vi "OCU_Main.vi"() -> ()   [LabVIEW 2013]
doc: "To be executed on the Opperator Control Unit (laptop), which communicates to a variety of platforms for the sailbot boat to send missions to complete, override commands, and to monitor the status of the boat and parts of the code run on it. It should be run in parallel with \"Main.vi\" in the cRIO code foler. \n\nCreaded by Victoria Coleman and Elizabeth Mahon (03/14)"
uses:
  cRIO_Code/Data/TypeDefs/MissionTypeControl.ctl
  cRIO_Code/Data/TypeDefs/UTM Location.ctl
  cRIO_Code/Data/TypeDefs/MissionDescription.ctl
  cRIO_Code/Data/TypeDefs/MainsailPositionIndicator.ctl
  cRIO_Code/Data/TypeDefs/JibPositionIndicator.ctl
  cRIO_Code/Data/TypeDefs/Rudder Set Suggestions.ctl
  cRIO_Code/Data/TypeDefs/OverrideMode.ctl
  cRIO_Code/Data/TypeDefs/Constants for OCU Tuning.ctl
  cRIO_Code/Data/TypeDefs/MotorSetup.ctl
  cRIO_Code/Data/TypeDefs/DynamixelSetupInfo.ctl
  TypeDef/map_list.ctl
  cRIO_Code/Data/TypeDefs/Sail Set Suggestions.ctl
  cRIO_Code/Data/TypeDefs/Sim_Wind_Heading.ctl
  cRIO_Code/Data/TypeDefs/Sim_Wind_Speed.ctl
  cRIO_Code/Logic/Classes/Missions/GenericMission/GenericMission.lvclass
  cRIO_Code/Data/TypeDefs/OverrideInformation.ctl
  cRIO_Code/Data/TypeDefs/Apparent Wind Point of Sail.ctl
  cRIO_Code/Data/TypeDefs/ObstacleDescription.ctl
  cRIO_Code/Logic/Classes/Obstacle/Obstacle.lvclass
  cRIO_Code/Data/TypeDefs/BoatType.ctl
  cRIO_Code/Logic/Classes/Waypoint/Waypoint.lvclass
  CommandMessages.ctl
  <vilib>/event_ctls.llb/eventvkey.ctl
  cRIO_Code/Logic/Classes/Missions/GoTo/GoTo.lvclass
  RIO-OCU_Comm/NetworkStreams/Writer/NetworkStreamWriter.lvclass
  RIO-OCU_Comm/NetworkStreams/Reader/NetworkStreamReader.lvclass
panel:
  in  "Do \"Initialize Me!\" Before running":enum32{"Initialize Me!", "Tuneable Constants"}(tab)
  in  "Boat Type":T1=enum."Damn Yankee"
  in  "Map":T2=enum."Olin"
  out "Writter\nConnected?":bool
  out "Reader\nConnected?":bool
  in  "OCU Tuning Constants":T3={"Motor Setting Constant"={"Main Dynamixel Set Data"={"Lower Winch Bound (deg)"=0.0, "Upper Winch Bound (deg)"=1000.0}, "Rudder Dynamixel Set Data"={"Lower Winch Bound (deg)"=30.0, "Upper Winch Bound (deg)"=90.0}, "Jib Dynamixel Set Data"={"Lower Winch Bound (deg)"=0.0, "Upper Winch Bound (deg)"=700.0}}, "Irons Range (deg)"=45.0}
  in  "Main Tab Structure":T6(tab)
  in  "Trace Path":bool=TRUE
  in  "Setting Missions with Map Internal Tab":T7(tab)
  in  "ClearMissionPOI":bool
  in  "CreateMission":bool
  in  "Mission Type":T8=enum."Drive to Waypoint"
  in  "Mission Points of Interest":T9[](array[typedef]) {"North" format="%#_10f"; "East" format="%#_8f"}
  in  "Tolerance (m)":dbl=10.0
  in  "Duration (s)\n[For in-box mission]":dbl=-1.0
  in  "Timeout (s)":dbl=-1.0
  out "Current Missions str":T10[](array[typedef]) {"Points of Interest"."North" format="%#_10f"; "Points of Interest"."East" format="%#_8f"}
  in  "ID# To Delete (miss)":u16
  in  "DeleteMission":bool
  out "# of Missions":i32
  in  "ClearObstaclePOI":bool
  out "# of Obstacles":i32
  in  "DeleteObstacle":bool
  in  "ID# To Delete (obs)":u16
  in  "Obstacle Points of Interest":T9[](array[typedef]) {"North" format="%#_10f"; "East" format="%#_8f"}
  in  "CreateObstacle":bool
  out "Current Obstacles":T11[](array[typedef]) {"Obstacle Array"."North" format="%#_10f"; "Obstacle Array"."East" format="%#_8f"}
  out "Robot Location":T9 {"North" format="%#_10f"; "East" format="%#_8f"}
  out "Rudder Setpoint":T12 min=-0.95 max=0.95 scale=1.0..-1.0
  out "BoatSpeed":dbl
  out "Abs Wind Direction":dbl(knob)
  out "Main":T13
  out "Jib":T14
  out "BoatDirection":dbl(knob)
  out "Rudder\noverridden?":bool
  out "Sail\noverridden?":bool
  out "RelWindDirection":T15 scale=0.0..360.0 scale format="%4d"
  in  "Sim_Wind_Heading":T16
  in  "Sim_Wind_Speed":T17
  out "Set Mission with Map":T18(plugin-control)
  in  "Clear Trace":bool
  in  "Plot Obstacles":bool=TRUE
  out "Sending IDs?":bool
  out "Manual Control Map":T18(plugin-control)
  in  "Main":T13
  in  "Jib":T14
  in  "Manual Rudder Setpoint":T12 min=-0.95 max=0.95 scale=1.0..-1.0
  in  "OverrideMode":T19
  out "Reset missions?":bool=TRUE
  out "Missions from Main":refnum<class "GenericMission.lvclass">[](array[class])
  out "Current Obstacles":refnum<class "Obstacle.lvclass">[](array[class])
  out "Current Missions":refnum<class "GenericMission.lvclass">[](array[class])
  out "Finished Missions":refnum<class "GenericMission.lvclass">[](array[class])
  out "Map display loop counter":i32
  out "User input loop counter":i32
  out "Desired Heading":dbl
  out "Abs Wind Direction":dbl(knob)
  out "Rel Wind Direction":dbl(knob)
  out "Sail Positions":T20 {"MainSailSuggestion" min=0.0 max=1.0; "JibSailSuggestion" min=0.0 max=1.0}
  out "Rudder Setpoint":T12 min=-0.95 max=0.95 scale=1.0..-1.0
  out "BoatDirection":dbl
  out "Override info":T21 {"SailSetting"."MainSailSuggestion" min=0.0 max=1.0; "SailSetting"."JibSailSuggestion" min=0.0 max=1.0; "Rudder Setpoint" min=-0.95 max=0.95 scale=1.0..-1.0}
  out "Final error out":errorcluster
  out "Intermediate\nWaypoints":refnum<class "Waypoint.lvclass">[](array[class])
  in  "stop":bool
  # "RUN MAIN.VI FIRST. SERIOUSLY"
  # "Add the \"Local GPS\" section of the old code so that we can grab GPS points from the boat and save them as waypoints or points of interest."
  # "If you forgot to set the boat type, you must restart the code"
  # "Reorganize this section, maybe split the cluster up"
  # "# of Waypoints Total [implement this]"
  # "# of Waypoints Left [implement this]"
  # "Log Message [important that we implement this one]"
  # "This is where you should be able to clilck the map and set a waypoint. Look in the [Mission Map] [Mission Edit]tab in the old OCU\n(\\Software\\0-OCU\\0 Code\\0 OCU.vi)\nand check out how they set up and documented the point and click operation.\nEric, 4/5/14"
  # "Add Load MDF, Save MDF, and Clear Mission functionality. Clear missions would clear all current missions. Look at old OCU for examples"
  # "This is where you should be able to clilck the map and set a waypoint. Look in the [Mission Map] [Mission Edit]tab in the old OCU\n(\\Software\\0-OCU\\0 Code\\0 OCU.vi)\nand check out how they set up and documented the point and click operation.\nEric, 4/5/14"
  # "Add Load ODF, Save ODF, and Clear Mission functionality. Clear missions would clear all current missions. Look at old OCU for examples"
  # "Look in the [Mission Map][Monitering]tab in the old OCU\n(\\Software\\0-OCU\\0 Code\\0 OCU.vi)\nand check out how they displayed the boat information during runtime. Try and make the indicators pretty and try to give only critical information \n\nEric, 4/5/14"
  # "Boat Direction\nis in \"math\"\n0E, CCW\nincrease"
  # "Abs Wind\nis in \"math\"\n0E, CCW\nincrease"
  # "Set wind speed"
  # "Set water current speed"
  # "Look in the lower right of the old OCU\n(\\Software\\0-OCU\\0 Code\\0 OCU.vi)\nand check out how they tweaked the simulator during runtime. Do this later.\n\nEric, 4/5/14"
  # "Set boat position"
  # "KEY MAPPINGS TO ACTUATOR MOVEMENT:\n\n\"Up\" -- Main out    |  \"Page Down\" -- Jib out\n\"Down\" -- Main in  |  \"Right\" -- Jib in\n\n\"Page Up\" -- rudder right\n\"Left\" -- rudder left"
  # "PUT MAP HERE"
  # "Check out the Manual Mission Input in the bottom left of the old code: (\\Software\\0-OCU\\0 Code\\0 OCU.vi)"
  # "PUT ALL THE BOAT DATA HERE\nLook at the Detailed Telemetry section of the old OCU for inspiration on how to organize information (\\Software\\0-OCU\\0 Code\\0 OCU.vi)"
  # "These guys need to be kept even though they aren't human readable, they're used for probing and data passage"
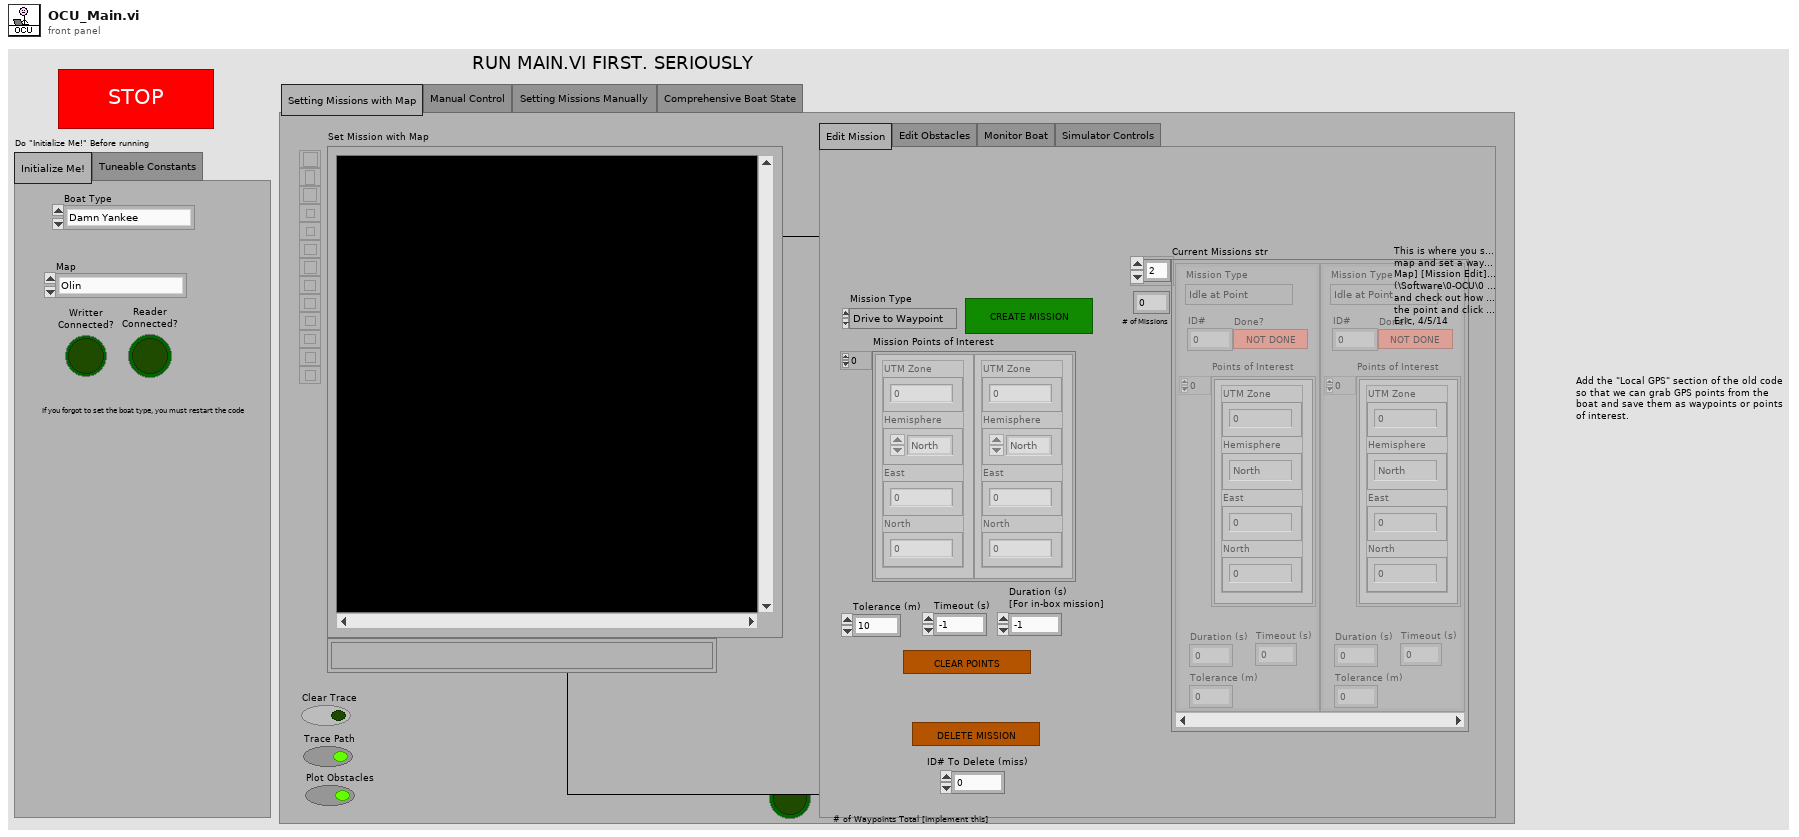
[diagram p1: front panel]
types:
  T1 = typedef "BoatType.ctl" = enum16{"Blackbody Radiation", "ReadLog", "Little boats", "Damn Yankee"}
  T2 = typedef "map_list.ctl" = enum16{"Grid", "Olin"}
  T3 = typedef "Constants for OCU Tuning.ctl" = cluster{"Motor Setting Constant":T4, "Irons Range (deg)":dbl}
  T4 = typedef "MotorSetup.ctl" = cluster{"Main Dynamixel Set Data":T5, "Rudder Dynamixel Set Data":T5, "Jib Dynamixel Set Data":T5}
  T5 = typedef "DynamixelSetupInfo.ctl" = cluster{"Lower Winch Bound (deg)":dbl, "Upper Winch Bound (deg)":dbl}
  T6 = enum32{"Setting Missions with Map", "Manual Control", "Setting Missions Manually ", "Comprehensive Boat State"}
  T7 = enum32{"Edit Mission", "Edit Obstacles", "Monitor Boat", "Simulator Controls"}
  T8 = typedef "MissionTypeControl.ctl" = enum16{"Idle at Point", "Drive to Waypoint", "Round Buoy to Port", "Round Buoy to Starboard", "Pass Between Buoys", "Station Keeping"}
  T9 = typedef "UTM Location.ctl" = cluster{"UTM Zone":dbl, "Hemisphere":enum16{"North", "South"}, "East":dbl, "North":dbl}
  T10 = typedef "MissionDescription.ctl" = cluster{"Duration (s)":dbl, "Timeout (s)":dbl, "Tolerance (m)":dbl, "Mission Type":T8, "Points of Interest":T9[], "ID#":i32, "Done?":bool}
  T11 = typedef "ObstacleDescription.ctl" = cluster{"ID#":i32, "Obstacle Array":T9[]}
  T12 = typedef "Rudder Set Suggestions.ctl" = dbl
  T13 = typedef "MainsailPositionIndicator.ctl" = dbl
  T14 = typedef "JibPositionIndicator.ctl" = dbl
  T15 = typedef "Apparent Wind Point of Sail.ctl" = dbl
  T16 = typedef "Sim_Wind_Heading.ctl" = dbl
  T17 = typedef "Sim_Wind_Speed.ctl" = dbl
  T18 = typedef "IMAQ Image.ctl" = refnum<image>
  T19 = typedef "OverrideMode.ctl" = enum16{"None", "Rudder", "Sails", "Both"}
  T20 = typedef "Sail Set Suggestions.ctl" = cluster{"MainSailSuggestion":dbl, "JibSailSuggestion":dbl}
  T21 = typedef "OverrideInformation.ctl" = cluster{"OverrideMode":T19, "SailSetting":T20, "Rudder Setpoint":T12, "Sim_Wind_Speed":dbl, "Sim_Wind_Heading":dbl}
  T22 = typedef "mission_arrays.ctl" = cluster{"# of Missions":i32, "Readable Missions":T10[], "Mission array":refnum<class "GenericMission.lvclass">[]}
  T23 = typedef "obstacle_arrays.ctl" = cluster{"# of Obstacles":i32, "Obstacle array":refnum<class "Obstacle.lvclass">[], "Readable Obstacles":T11[]}
  T24 = typedef "map_metadata.ctl" = cluster{"Meters/pixel":dbl, "Top Left Pixel UTM":T9, "Bottom Right Pixel UTM":T9}
  T25 = typedef "CommandMessages.ctl" = enum16{"Pass", "OverrideMode", "Add mission", "Delete mission", "Add obstacle", "Delete obstacle", "Change constants", "Check mission ID", "Check obstacle ID"}
  T26 = typedef "eventvkey.ctl" = enum16{"ASCII", "Enter", "Return", "Shift", "Ctrl", "Alt", "Cmd", "Opt", "Caps", "NumLock", "Clear", "Break", "Up", "Down", "Left", "Right", "Insert", "Delete", "Home", "End", "PageUp", "PageDown", "Escape", "Help", "Pause", "ScrollLock", "F1", "F2", "F3", "F4", "F5", "F6", "F7", "F8", "F9", "F10", "F11", "F12", "F13", "F14", "F15", "F16", "F17", "F18", "F19", "F20", "F21", "F22", "F23", "F24", "Play", "VolumeUp", "VolumeDown", "Mute", "Two Byte Char"}
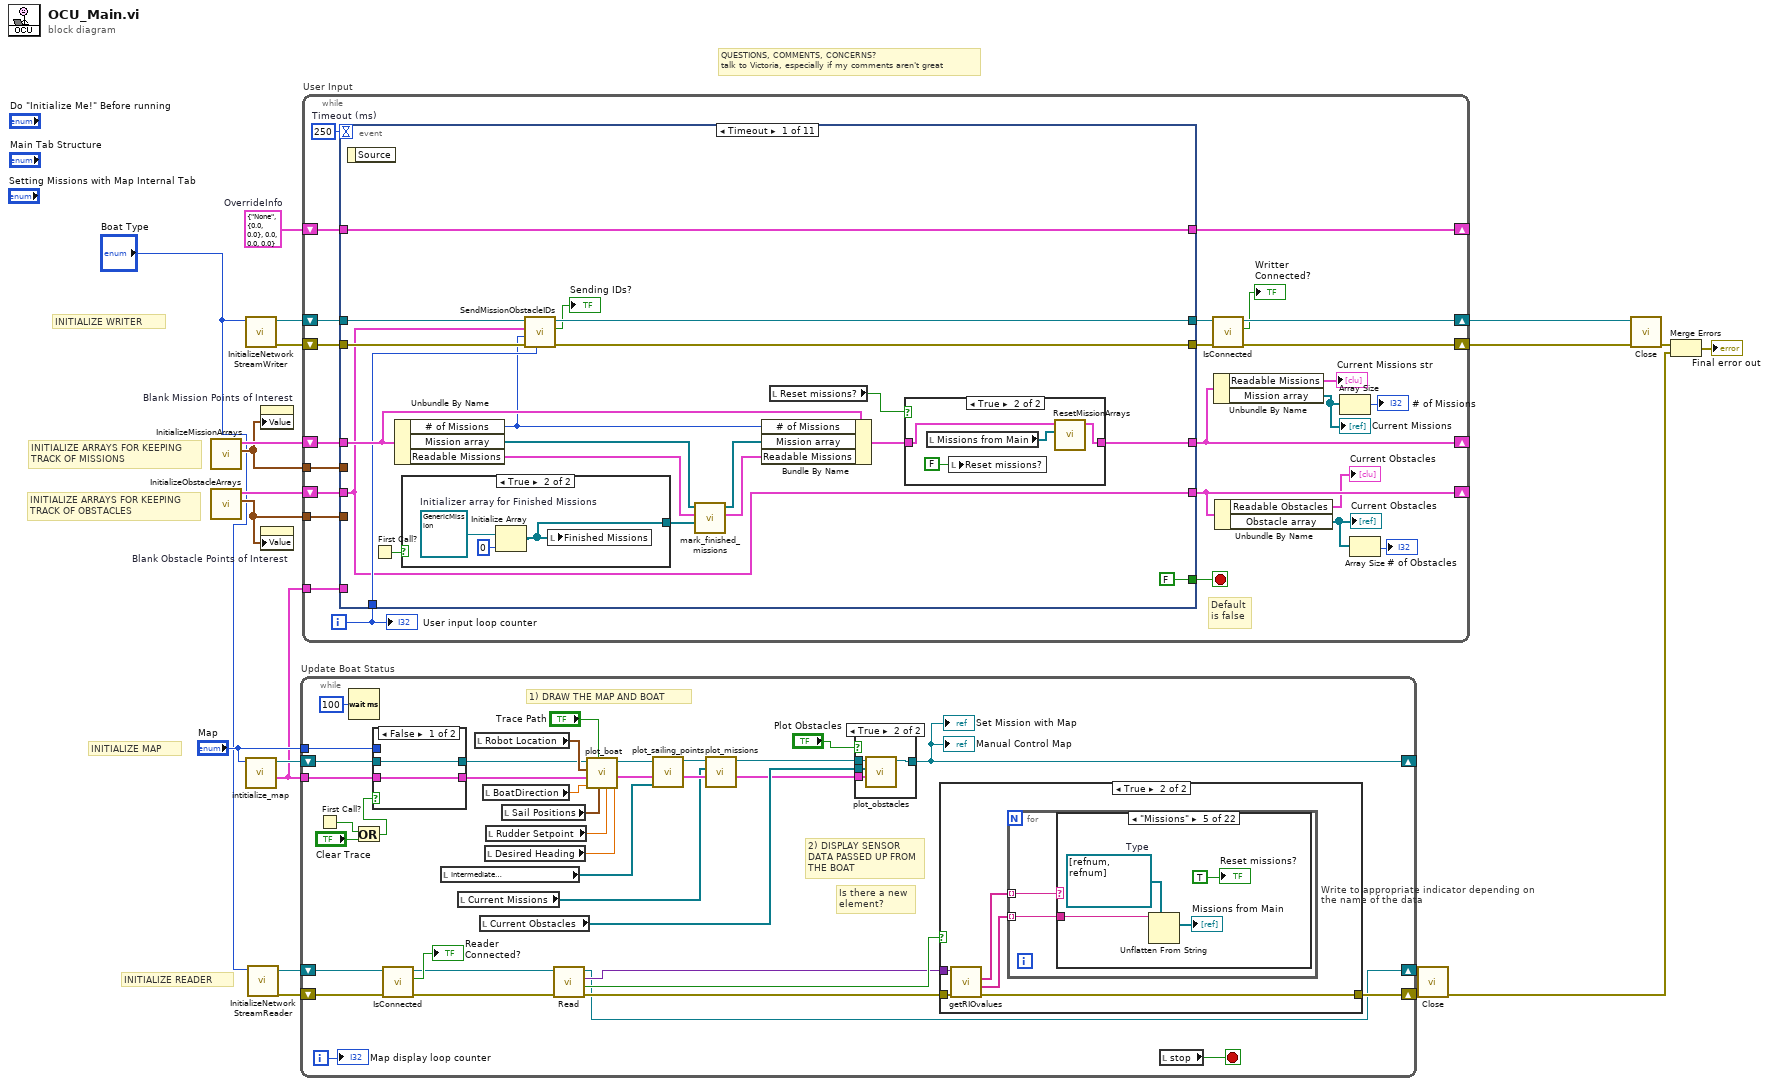
[diagram p0: block diagram]
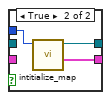
[diagram p3: hidden frame]
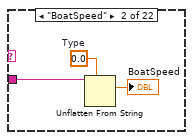
[diagram p6: hidden frame]
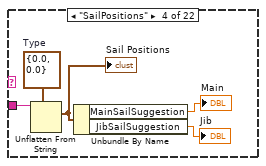
[diagram p8: hidden frame]
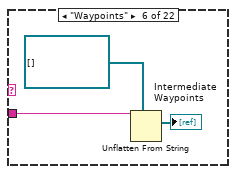
[diagram p9: hidden frame]
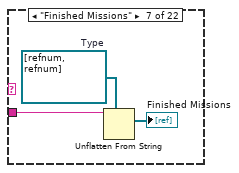
[diagram p10: hidden frame]
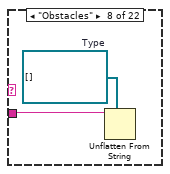
[diagram p11: hidden frame]
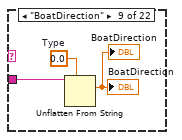
[diagram p12: hidden frame]
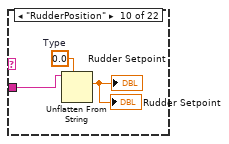
[diagram p13: hidden frame]
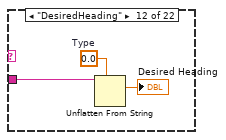
[diagram p15: hidden frame]
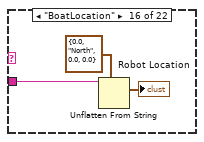
[diagram p19: hidden frame]
diagram:
  w6 = T21 {"OverrideMode"=enum."None", "SailSetting"={"MainSailSuggestion"=0.0, "JibSailSuggestion"=0.0}, "Rudder Setpoint"=0.0, "Sim_Wind_Speed"=0.0, "Sim_Wind_Heading"=0.0}  # OverrideInfo
  # "INITIALIZE ARRAYS FOR KEEPING TRACK OF OBSTACLES"
  # "INITIALIZE WRITER"
  # "INITIALIZE ARRAYS FOR KEEPING TRACK OF MISSIONS"
  # "INITIALIZE MAP"
  # "INITIALIZE READER"
  # "QUESTIONS, COMMENTS, CONCERNS? \ntalk to Victoria, especially if my comments aren't great"
  n1 = call "InitializeMissionArrays.vi"() -> ("Mission Points of Interest"=w2:T9[], "Initialized Mission Arrays"=w20:T22)  [unwired: 10 in]
  n2 = call "InitializeObstacleArrays.vi"() -> ("Obstacle Points of Interest"=w3:T9[], "Obstacle Arrays Cluster"=w4:T23)  [unwired: 10 in]
  n3 = call "InitializeNetworkStreamWriter.vi"("Boat Type"="Boat Type") -> ("error out"=w17:errorcluster, "NetworkStreamWriter out"=w16:refnum<class "NetworkStreamWriter.lvclass">)  [unwired: 9 in]
  n4 = call "intitialize_map.vi"("Map"="Map") -> ("MapDistanceInfo"=w5:T24, "Map Image Out"=w13:T18)  [unwired: 9 in]
  n5 = call "InitializeNetworkStreamReader.vi"("Boat Type"="Boat Type") -> ("error out"=w11:errorcluster, "NetworkStreamReader out"=w12:refnum<class "NetworkStreamReader.lvclass">)  [unwired: 9 in]
  n6 = property on="Blank Mission Points of Interest" class="Arr (strict)"("Value"=w2) -> ()  [unwired: 2 in, 2 out]
  n7 = property on="Blank Obstacle Points of Interest" class="Arr (strict)"("Value"=w3) -> ()  [unwired: 2 in, 2 out]
  n8 = while "Update Boat Status" {
    shift-right: [w47] -> w15
    shift-left: w12 -> [w57]
    shift-right: [w53] -> w14
    shift-left: w11 -> [w56]
    tunnel: w5 -> [w42]
    tunnel: "Map" -> [w44]
    shift-right: [w29] -> _
    shift-left: w13 -> [w45]
    i -> [w43]
    stop <- w58 stop-if-true
    # "Is there a new element?"
    # "2) DISPLAY SENSOR DATA PASSED UP FROM THE BOAT"
    # "1) DRAW THE MAP AND BOAT"
    n9 = First Call?() -> (First Call?: T/F=w32:bool)
    n10 = Wait (ms)(milliseconds to wait=u32 100) -> ()  [unwired: 1 out]
    n11 = Or(x=w32, y="Clear Trace") -> (x .or. y?=w31:bool)
    n12 = case shown="False" w31 {
      tunnel: w45 -> [w65 _]
      tunnel: [w65 w66] -> w34
      tunnel: w42 -> [w64 _]
      tunnel: [w64 w67] -> w35
      tunnel: w44 -> [_ w68]
      frame False {
      }
      frame True {
        n13 = call "intitialize_map.vi"("Map"=w68) -> ("MapDistanceInfo"=w67:T24, "Map Image Out"=w66:T18)  [unwired: 9 in]
      }
    }
    n14 = call "IsConnected.vi"("error in (no error)"=w56, "NetworkStreamReader in"=w57) -> ("error out"=w51:errorcluster, "Connected?"=→"Reader\nConnected?":bool, "NetworkStreamReader out"=w52:refnum<class "NetworkStreamReader.lvclass">)  [unwired: 7 in]
    n15 = local read "Intermediate\nWaypoints"() -> (w26:refnum<class "Waypoint.lvclass">[])
    n16 = local read "Current Missions"() -> (w21:refnum<class "GenericMission.lvclass">[])
    n17 = local read "Robot Location"() -> (w38:T9)
    n18 = local read "Current Obstacles"() -> (w28:refnum<class "Obstacle.lvclass">[])
    n19 = local read "BoatDirection"() -> (w40:dbl)
    n20 = local read "Desired Heading"() -> (w30:dbl)
    n21 = local read "Rudder Setpoint"() -> (w39:T12)
    n22 = local read "Sail Positions"() -> (w41:T20)
    n23 = call "Read.vi"("error in (no error)"=w51, "NetworkStreamReader in"=w52) -> ("error out"=w50:errorcluster, "New element?"=w49:bool, "element"=w48:variant, "NetworkStreamReader out"=w47:refnum<class "NetworkStreamReader.lvclass">)  [unwired: 5 in, 1 out]
    n24 = call "plot_boat.vi"("Desired Heading"=w30, "Rudder Setpoint"=w39, "Sail Setpoints"=w41, "Trace Path"="Trace Path", "Heading"=w40, "MapDistanceInfo"=w35, "UTM Location"=w38, "Map in"=w34) -> ("MapDistanceInfo OUT"=w36:T24, "Map Out"=w37:T18)  [unwired: 1 in, 1 out]
    n25 = call "plot_sailing_points.vi"("Intermediate\nWaypoints"=w26, "MapDistanceInfo"=w36, "Map in"=w37) -> ("MapDistanceInfo OUT"=w25:T24, "Map Out"=w23:T18)  [unwired: 6 in, 1 out]
    n26 = call "plot_missions.vi"("MapDistanceInfo"=w25, "Missions"=w21, "Map in"=w23) -> ("MapDistanceInfo OUT"=w24:T24, "Map Out"=w22:T18)  [unwired: 6 in, 1 out]
    n27 = case shown="True" "Plot Obstacles" {
      tunnel: w22 -> [w59 w63]
      tunnel: [w59 w62] -> w29
      tunnel: w24 -> [_ w61]
      tunnel: w28 -> [_ w60]
      frame False {
      }
      frame True {
        n28 = call "plot_obstacles.vi"("MapDistanceInfo"=w61, "Current Obstacles"=w60, "Map in"=w63) -> ("Map Out"=w62:T18)  [unwired: 7 in, 1 out]
      }
    }
    "Set Mission with Map" <- w29
    "Manual Control Map" <- w29
    n29 = case shown="True" w49 {
      tunnel: [w69 w72] -> w53
      tunnel: w50 -> [w69 w71]
      tunnel: w48 -> [_ w70]
      frame False {
      }
      frame True {
        n30 = call "getRIOvalues.vi"("error in"=w71, "element"=w70) -> ("error out"=w72:errorcluster, "data"=w73:string[], "names"=w74:string[])  [unwired: 7 in]
        n31 = for "Write to appropriate indicator depending on the name of the data" {
          tunnel: w74 -> [w76] mode=indexing
          tunnel: w73 -> [w75] mode=indexing
          n32 = case shown="\"Missions\"" w76 {
            tunnel: w75 -> [_ w77 _ w84 w87 w91 w94 w95 w99 w102 _ w103 _ _ _ w108 _ _ _ w110 w114 _]
            frame Default {
              # "unknown name"
            }
            frame "BoatSpeed" {
              w79 = 0.0  # Type
              n33 = Unflatten From String(type=w79, binary string=w77) -> (value=→"BoatSpeed":dbl)  [unwired: 3 in, 2 out]
            }
            frame "WindSpeed" {
            }
            frame "SailPositions" {
              w83 = T20 {"MainSailSuggestion"=0.0, "JibSailSuggestion"=0.0}  # Type
              n34 = Unflatten From String(type=w83, binary string=w84) -> (value=w82:T20)  [unwired: 3 in, 2 out]
              "Sail Positions" <- w82
              n35 = Unbundle By Name(w82) -> ("MainSailSuggestion"=→"Main":dbl, "JibSailSuggestion"=→"Jib":dbl)
            }
            frame "Missions" {
              w88 = refnum<class "GenericMission.lvclass">[] [refnum, refnum]  # Type
              n36 = Unflatten From String(type=w88, binary string=w87) -> (value=→"Missions from Main":refnum<class "GenericMission.lvclass">[])  [unwired: 3 in, 2 out]
              "Reset missions?" <- TRUE
            }
            frame "Waypoints" {
              n37 = Unflatten From String(type=refnum<class "Waypoint.lvclass">[] [] ("elements"), binary string=w91) -> (value=→"Intermediate\nWaypoints":refnum<class "Waypoint.lvclass">[])  [unwired: 3 in, 2 out]
            }
            frame "Finished Missions" {
              w93 = refnum<class "GenericMission.lvclass">[] [refnum, refnum]  # Type
              n38 = Unflatten From String(type=w93, binary string=w94) -> (value=→"Finished Missions":refnum<class "GenericMission.lvclass">[])  [unwired: 3 in, 2 out]
            }
            frame "Obstacles" {
              w96 = refnum<class "Obstacle.lvclass">[] []  # Type
              n39 = Unflatten From String(type=w96, binary string=w95) -> ()  [unwired: 3 in, 3 out]
            }
            frame "BoatDirection" {
              w98 = 0.0  # Type
              n40 = Unflatten From String(type=w98, binary string=w99) -> (value=→"BoatDirection" →"BoatDirection":dbl)  [unwired: 3 in, 2 out]
            }
            frame "RudderPosition" {
              w101 = T12 0.0  # Type
              n41 = Unflatten From String(type=w101, binary string=w102) -> (value=→"Rudder Setpoint" →"Rudder Setpoint":T12)  [unwired: 3 in, 2 out]
            }
            frame "SimWindSpeed(m/s)" {
            }
            frame "DesiredHeading" {
              w105 = 0.0  # Type
              n42 = Unflatten From String(type=w105, binary string=w103) -> (value=→"Desired Heading":dbl)  [unwired: 3 in, 2 out]
            }
            frame "RudderForce" {
            }
            frame "BatteryVoltage" {
            }
            frame "StayForces" {
            }
            frame "BoatLocation" {
              n43 = Unflatten From String(type=T9 {"UTM Zone"=0.0, "Hemisphere"=enum."North", "East"=0.0, "North"=0.0} ("UTM Location"), binary string=w108) -> (value=→"Robot Location":T9)  [unwired: 3 in, 2 out]
            }
            frame "Pitch" {
            }
            frame "Roll" {
            }
            frame "RateOfTurn" {
            }
            frame "RelWindDirection" {
              w111 = 0.0  # Type
              n44 = Unflatten From String(type=w111, binary string=w110) -> (value=→"Rel Wind Direction" →"RelWindDirection":dbl)  [unwired: 3 in, 2 out]
            }
            frame "AbsWindDirection" {
              w113 = 0.0  # Type
              n45 = Unflatten From String(type=w113, binary string=w114) -> (value=→"Abs Wind Direction" →"Abs Wind Direction":dbl)  [unwired: 3 in, 2 out]
            }
            frame "DynamixelTorques" {
            }
          }
        }
      }
    }
    n46 = local read "stop"() -> (w58:bool)
    "Map display loop counter" <- w43
  }
  n47 = while "User Input" {
    shift-right: [w124] -> _
    shift-left: w20 -> [w139]
    shift-right: [w132] -> w18
    shift-left: w17 -> [w136]
    shift-right: [w133] -> w19
    shift-left: w16 -> [w135]
    shift-right: [w130] -> _
    shift-left: w6 -> [w129]
    tunnel: w5 -> [w127]
    tunnel: w2 -> [w126]
    tunnel: w3 -> [w121]
    shift-right: [w119] -> _
    shift-left: w4 -> [w120]
    i -> [w115]
    stop <- w137 stop-if-true
    w125 = 250  # Timeout (ms)
    # "Default is false"
    n48 = event shown="[0] Timeout" {
      selector: _ -> [_ _ _ _ _ _ _ _ _ _ _]
      dyn-events: _ -> [_ _ _ _ _ _ _ _ _ _ _]
      timeout: w125 -> [_ _ _ _ _ _ _ _ _ _ _]
      tunnel: w139 -> [w155 w171 w189 w211 w236 w255 w262 w278 w290 w338 w369]
      tunnel: [FALSE TRUE FALSE _ FALSE _ _ _ _ _ _] -> w137
      tunnel: [w144 w170 w182 w212 w245 w253 w259 w273 w293 w336 w367] -> w128
      tunnel: w135 -> [w149 w173 w187 w215 w243 w251 w258 w276 w301 w357 w373]
      tunnel: w136 -> [w150 w170 w186 w214 w244 w254 w261 w281 w299 w347 w374]
      tunnel: [w145 w173 w185 w213 w242 w252 w258 w276 w300 w356 w372] -> w134
      tunnel: [w158 w172 w184 w218 w241 w256 w257 w279 w291 w342 w370] -> w130
      tunnel: w129 -> [w158 w172 w184 w218 w241 w256 w257 w279 w292 w355 w370]
      tunnel: w127 -> [_ _ _ _ _ _ _ w282 _ _ _]
      tunnel: w126 -> [_ _ w183 _ _ _ w265 _ _ _ _]
      tunnel: [w141 w171 w176 w211 w240 w255 w262 w278 w290 w338 w369] -> w124
      tunnel: w121 -> [_ _ _ w210 _ _ w264 _ _ _ _]
      tunnel: w120 -> [w147 w169 w175 w209 w239 w248 w263 w277 w289 w337 w368]
      tunnel: [w147 w169 w175 w208 w239 w247 w263 w277 w289 w337 w368] -> w119
      tunnel: w115 -> [w148 _ _ _ _ _ _ _ _ _ _]
      event Timeout {
        n49 = event-data() -> ()  [unwired: 1 in, 1 out]
        n50 = First Call?() -> (First Call?: T/F=w156:bool)
        n51 = Unbundle By Name(w155) -> ("# of Missions"=w146:i32, "Mission array"=w154:refnum<class "GenericMission.lvclass">[], "Readable Missions"=w153:T10[])
        n52 = case shown="True" w156 {
          tunnel: [w165 w166] -> w157
          frame False {
            n53 = local read "Finished Missions"() -> (w165:refnum<class "GenericMission.lvclass">[])
          }
          frame True {
            w168 = refnum<class "GenericMission.lvclass"> refnum  # Initializer array for Finished Missions
            n54 = Initialize Array(w168, 0 ("dimension size")) -> (w166:refnum<class "GenericMission.lvclass">[])
            n55 = local write "Finished Missions"(w166) -> ()
          }
        }
        n56 = call "SendMissionObstacleIDs.vi"("Loop counter"=w148, "error in (no error)"=w150, "# of Missions"=w146, "Obstacle Arrays Cluster"=w147, "NetworkStreamWriter in"=w149) -> ("error out"=w144:errorcluster, "Sending IDs?"=→"Sending IDs?":bool, "NetworkStreamWriter out"=w145:refnum<class "NetworkStreamWriter.lvclass">)  [unwired: 4 in]
        n57 = call "mark_finished_missions.vi"("Finished Missions"=w157, "Current Missions (human readable)"=w153, "Current Missions"=w154) -> (2:"Current Missions OUT"=w152:T10[], 3:"Current Missions OUT"=w151:refnum<class "GenericMission.lvclass">[])  [unwired: 7 in]
        n58 = Bundle By Name(cluster=w155, "# of Missions"=w146, "Mission array"=w151, "Readable Missions"=w152) -> (w142:T22)
        n59 = local read "Reset missions?"() -> (w143:bool)
        n60 = case shown="True" w143 {
          tunnel: w142 -> [w160 w163]
          tunnel: [w160 w162] -> w141
          frame False {
          }
          frame True {
            n61 = local read "Missions from Main"() -> (w161:refnum<class "GenericMission.lvclass">[])
            n62 = local write "Reset missions?"(FALSE ("Reset missions?")) -> ()
            n63 = call "ResetMissionArrays.vi"("Mission Array Replacement"=w161, "Mission Arrays"=w163) -> ("Mission Arrays"=w162:T22)  [unwired: 9 in]
          }
        }
      }
      event "stop": Value Change {
        # "Putting the button in here keeps the code from breaking, leave it here :)\nHas to do with how event structures work"
        n64 = event-data() -> ()  [unwired: 1 in, 2 out]
      }
      event "CreateMission": Value Change {
        n65 = event-data() -> ("OldVal"=w177:bool)  [unwired: 1 in]
        n66 = Array Size(array="Mission Points of Interest") -> (size(s)=w180:i32)
        n67 = Not Equal To 0?(x=w180) -> (x != 0?=w178:bool)
        n68 = And(x=w177, y=w178) -> (x .and. y?=w179:bool)
        n69 = case shown="False" w179 {
          tunnel: w189 -> [w190 w200]
          tunnel: [w190 w194] -> w176
          tunnel: [w192 w202] -> w182
          tunnel: w187 -> [w191 w205]
          tunnel: w186 -> [w192 _]
          tunnel: [w191 w203] -> w185
          tunnel: w183 -> [_ w193]
          tunnel: "Mission Points of Interest" -> [_ w199]
          frame False {
          }
          frame True {
            # "send created message to Forebrain"
            n70 = property on="Mission Points of Interest" class="Arr (strict)"("Value"=w193) -> ()  [unwired: 2 in, 2 out]
            n71 = call "CreateNewMissions.vi"("Timeout (s)"="Timeout (s)", "Duration (s)\n[For in-box mission]"="Duration (s)\n[For in-box mission]", "Tolerance (m)"="Tolerance (m)", "Mission Type"="Mission Type", "Points of Interest"=w199, "Initialized Mission Arrays"=w200) -> ("New Mission OUT"=w195:refnum<class "GenericMission.lvclass">, "Mission Array Cluster"=w194:T22)  [unwired: 4 in]
            n72 = Flatten To String(anything=w195) -> (data string=w204:string, error out=w201:errorcluster)  [unwired: 3 in, 1 out]
            n73 = call "MapAndWrite.vi"("error in (no error)"=w201, "String_Cast_of_Info"=w204, "Commands"=CommandMessages."Add mission", "NetworkStreamWriter in"=w205) -> ("error out"=w202:errorcluster, "NetworkStreamWriter out"=w203:refnum<class "NetworkStreamWriter.lvclass">)  [unwired: 2 in]
          }
        }
      }
      event "CreateObstacle": Value Change {
        n74 = event-data() -> ("OldVal"=w219:bool)  [unwired: 1 in]
        n75 = Array Size(array="Obstacle Points of Interest") -> (size(s)=w221:i32)
        n76 = Not Equal To 0?(x=w221) -> (x != 0?=w220:bool)
        n77 = And(x=w219, y=w220) -> (x .and. y?=w217:bool)
        n78 = case shown="True" w217 {
          tunnel: "Obstacle Points of Interest" -> [_ w229]
          tunnel: w215 -> [w224 w230]
          tunnel: w214 -> [w223 _]
          tunnel: [w224 w232] -> w213
          tunnel: [w223 w231] -> w212
          tunnel: w210 -> [_ w225]
          tunnel: w209 -> [w222 w228]
          tunnel: [w222 w227] -> w208
          frame False {
          }
          frame True {
            # "send created message to Forebrain"
            n79 = property on="Obstacle Points of Interest" class="Arr (strict)"("Value"=w225) -> ()  [unwired: 2 in, 2 out]
            n80 = call "CreateNewObstacles.vi"("Obstacle Arrays Cluster IN"=w228, "Points of Interest"=w229) -> ("Obstacle Arrays Cluster OUT"=w227:T23, "New Obstacle OUT"=w226:refnum<class "Obstacle.lvclass">)  [unwired: 8 in]
            n81 = Flatten To String(anything=w226) -> (data string=w234:string, error out=w233:errorcluster)  [unwired: 3 in, 1 out]
            n82 = call "MapAndWrite.vi"("error in (no error)"=w233, "String_Cast_of_Info"=w234, "Commands"=CommandMessages."Add obstacle", "NetworkStreamWriter in"=w230) -> ("error out"=w231:errorcluster, "NetworkStreamWriter out"=w232:refnum<class "NetworkStreamWriter.lvclass">)  [unwired: 2 in]
          }
        }
      }
      event "DeleteMission": Value Change {
        n83 = event-data() -> ("OldVal"=w238:bool)  [unwired: 1 in]
        n84 = call "DeleteMission.vi"("OldVal"=w238, "ID# To Delete (miss)"="ID# To Delete (miss)", "error in (no error)"=w244, "Initialized Mission Arrays in"=w236, "NetworkStreamWriter in"=w243) -> ("error out"=w245:errorcluster, "Initialized Mission Arrays out"=w240:T22, "NetworkStreamWriter out"=w242:refnum<class "NetworkStreamWriter.lvclass">)  [unwired: 4 in]
      }
      event "DeleteObstacle": Value Change {
        n85 = event-data() -> ("OldVal"=w249:bool)  [unwired: 1 in]
        n86 = call "DeleteObstacle.vi"("OldVal"=w249, "ID# To Delete (miss)"="ID# To Delete (obs)", "error in (no error)"=w254, "Obstacle Arrays Cluster IN"=w248, "NetworkStreamWriter in"=w251) -> ("error out"=w253:errorcluster, "Obstacle Arrays Cluster OUT"=w247:T23, "NetworkStreamWriter out"=w252:refnum<class "NetworkStreamWriter.lvclass">)  [unwired: 4 in]
      }
      event "ClearObstaclePOI", "ClearMissionPOI": Value Change {
        n87 = event-data() -> ()  [unwired: 1 in, 2 out]
        n88 = property on="Setting Missions with Map Internal Tab" class="TabCtl (strict)"(error in=w261) -> (error out=w260:errorcluster, "Value"=w266:T7)  [unwired: 1 in, 1 out]
        n89 = case shown="\"Edit Mission\", Default" w266 {
          tunnel: w265 -> [w269 _]
          tunnel: w264 -> [_ w272]
          tunnel: w260 -> [w268 w271]
          tunnel: [w267 w270] -> w259
          frame "Edit Mission", Default {
            n90 = property on="Mission Points of Interest" class="Arr (strict)"(error in=w268, "Value"=w269) -> (error out=w267:errorcluster)  [unwired: 1 in, 1 out]
          }
          frame "Edit Obstacles" {
            n91 = property on="Obstacle Points of Interest" class="Arr (strict)"(error in=w271, "Value"=w272) -> (error out=w270:errorcluster)  [unwired: 1 in, 1 out]
          }
        }
      }
      event "Set Mission with Map": Mouse Up {
        n92 = event-data() -> ()  [unwired: 1 in, 3 out]
        n93 = property on="Set Mission with Map" class="ImageControl"(error in=w281) -> (error out=w273:errorcluster, "Last Mouse Position"=w280:cluster{"X":i32, "Y":i32})  [unwired: 1 in, 1 out]
        n94 = call "ImageUTMPosition.vi"("Pixel Coordinates"=w280, "MapDistanceInfo"=w282) -> ("output cluster"=w274:T9)  [unwired: 9 in]
        n95 = property on="Setting Missions with Map Internal Tab" class="TabCtl (strict)"() -> ("Value"=w275:T7)  [unwired: 2 in, 2 out]
        n96 = case shown="\"Edit Obstacles\"" w275 {
          tunnel: w274 -> [_ w283 w286]
          frame Default {
          }
          frame "Edit Mission" {
            n97 = property on="Mission Points of Interest" class="Arr (strict)"() -> ("Value"=w284:T9[])  [unwired: 2 in, 2 out]
            n98 = Build Array (concatenate)(w284, w283) -> (w285:T9[])
            n99 = property on="Mission Points of Interest" class="Arr (strict)"("Value"=w285) -> ()  [unwired: 2 in, 2 out]
          }
          frame "Edit Obstacles" {
            n100 = property on="Obstacle Points of Interest" class="Arr (strict)"() -> ("Value"=w287:T9[])  [unwired: 2 in, 2 out]
            n101 = Build Array (concatenate)(w287, w286) -> (w288:T9[])
            n102 = property on="Obstacle Points of Interest" class="Arr (strict)"("Value"=w288) -> ()  [unwired: 2 in, 2 out]
          }
        }
      }
      event Key Down; Key Repeat {
        n103 = event-data() -> ("VKey"=w295:T26)  [unwired: 1 in]
        n104 = local read "OverrideMode"() -> (w294:T19)
        n105 = case "Only if Special key pressed" shown="Default" w295 {
          selector: w295 -> [_ w312]
          tunnel: w301 -> [w304 w309]
          tunnel: [w304 w310] -> w300
          tunnel: w299 -> [w303 w311]
          tunnel: [w303 w307] -> w293
          tunnel: "Manual Rudder Setpoint" -> [_ w315]
          tunnel: "Jib" -> [_ w314]
          tunnel: "Main" -> [_ w313]
          tunnel: w294 -> [_ w308]
          tunnel: w292 -> [w302 w306]
          tunnel: [w302 w305] -> w291
          frame "ASCII" {
            # "No special key pressed :("
          }
          frame Default {
            n106 = case "Only executes of any actuators are in override mode" shown="Default" w308 {
              selector: w308 -> [_ w319]
              tunnel: w315 -> [_ w333]
              tunnel: w314 -> [_ w334]
              tunnel: w313 -> [_ w335]
              tunnel: w312 -> [_ w332]
              tunnel: w311 -> [w317 w331]
              tunnel: [w318 w327] -> w310
              tunnel: w309 -> [w318 w328]
              tunnel: [w317 w329] -> w307
              tunnel: w306 -> [w316 w326]
              tunnel: [w316 w321] -> w305
              frame "None" {
              }
              frame Default {
                # "KEY MAPPINGS TO ACTUATOR MOVEMENT:\n\"Page Up\" -- rudder right       |    \"Up\" -- Main out          |     \"Page Down\" -- Jib out\n\"Left\" -- rudder left                  |      \"Down\" -- Main in     |      \"Right\" -- Jib in"
                n107 = call "Write_NetworkStream_OCU_Override.vi"("VKey"=w332, "Mainsail Position"=w335, "Jib Position"=w334, "Rudder Setpoint"=w333, "error in (no error)"=w331, "OverrideMode"=w319) -> ("Main Position"=w323:T13, "Jib Position"=w324:T14, "Rudder Position"=w325:T12, "error out"=w330:errorcluster)  [unwired: 5 in, 1 out]
                n108 = Bundle By Name(cluster=w326, "OverrideMode"=w319, "SailSetting.MainSailSuggestion"=w323, "SailSetting.JibSailSuggestion"=w324, "Rudder Setpoint"=w325) -> (w321:T21)
                n109 = Flatten To String(anything=w321) -> (data string=w322:string)  [unwired: 3 in, 2 out]
                n110 = call "MapAndWrite.vi"("error in (no error)"=w330, "String_Cast_of_Info"=w322, "Commands"=CommandMessages."OverrideMode", "NetworkStreamWriter in"=w328) -> ("error out"=w329:errorcluster, "NetworkStreamWriter out"=w327:refnum<class "NetworkStreamWriter.lvclass">)  [unwired: 2 in]
              }
            }
          }
        }
      }
      event Value Change {
        # "Just an obscure key to make everything update (hackish solution to reuse vi)"
        n111 = event-data() -> ()  [unwired: 1 in, 2 out]
        n112 = local read "Manual Rudder Setpoint"() -> (w350:T12)
        n113 = local read "Jib"() -> (w351:T14)
        n114 = local read "OverrideMode"() -> (w348:T19)
        n115 = local read "Main"() -> (w352:T13)
        n116 = call "Write_NetworkStream_OCU_Override.vi"("VKey"=eventvkey."F24", "Mainsail Position"=w352, "Jib Position"=w351, "Rudder Setpoint"=w350, "error in (no error)"=w347, "OverrideMode"=w348) -> ("Main Position"=w345:T13, "Jib Position"=w344:T14, "Rudder Position"=w343:T12, "error out"=w346:errorcluster)  [unwired: 5 in, 1 out]
        n117 = Bundle By Name(cluster=w355, "OverrideMode"="OverrideMode", "Sim_Wind_Speed"="Sim_Wind_Speed", "Sim_Wind_Heading"="Sim_Wind_Heading", "SailSetting.MainSailSuggestion"=w345, "SailSetting.JibSailSuggestion"=w344, "Rudder Setpoint"=w343) -> (w342:T21)
        "Override info" <- w342
        n118 = case shown="\"None\", Default" "OverrideMode" {
          tunnel: [w361 FALSE ("Connected?") TRUE ("Connected?") w366] -> w341
          tunnel: [w361 TRUE ("Connected?") FALSE ("Connected?") w366] -> w340
          frame "None", Default {
            w361 = FALSE ("Connected?")
          }
          frame "Rudder" {
          }
          frame "Sails" {
          }
          frame "Both" {
            w366 = TRUE ("Connected?")
          }
        }
        "Rudder\noverridden?" <- w340
        "Sail\noverridden?" <- w341
        n119 = Flatten To String(anything=w342, error in (no error)=w346) -> (data string=w359:string, error out=w360:errorcluster)  [unwired: 2 in, 1 out]
        n120 = call "MapAndWrite.vi"("error in (no error)"=w360, "String_Cast_of_Info"=w359, "Commands"=CommandMessages."OverrideMode", "NetworkStreamWriter in"=w357) -> ("error out"=w336:errorcluster, "NetworkStreamWriter out"=w356:refnum<class "NetworkStreamWriter.lvclass">)  [unwired: 2 in]
      }
      event Value Change {
        n121 = event-data() -> ()  [unwired: 1 in, 2 out]
        n122 = Flatten To String(anything="OCU Tuning Constants", error in (no error)=w374) -> (data string=w376:string, error out=w375:errorcluster)  [unwired: 2 in, 1 out]
        n123 = call "MapAndWrite.vi"("error in (no error)"=w375, "String_Cast_of_Info"=w376, "Commands"=CommandMessages."Change constants", "NetworkStreamWriter in"=w373) -> ("error out"=w367:errorcluster, "NetworkStreamWriter out"=w372:refnum<class "NetworkStreamWriter.lvclass">)  [unwired: 2 in]
      }
    }
    n124 = call "IsConnected.vi"("error in (no error)"=w128, "NetworkStreamWriter in"=w134) -> ("error out"=w132:errorcluster, "Connected?"=→"Writter\nConnected?":bool, "NetworkStreamWriter out"=w133:refnum<class "NetworkStreamWriter.lvclass">)  [unwired: 7 in]
    n125 = Unbundle By Name(w124) -> ("Readable Missions"=→"Current Missions str":T10[], "Mission array"=w122:refnum<class "GenericMission.lvclass">[])
    "Current Missions" <- w122
    n126 = Unbundle By Name(w119) -> ("Readable Obstacles"=→"Current Obstacles":T11[], "Obstacle array"=w117:refnum<class "Obstacle.lvclass">[])
    "Current Obstacles" <- w117
    n127 = Array Size(array=w122) -> (size(s)=→"# of Missions":i32)
    n128 = Array Size(array=w117) -> (size(s)=→"# of Obstacles":i32)
    "User input loop counter" <- w115
  }
  n129 = call "Close.vi"("error in (no error)"=w14, "NetworkStreamReader in"=w15) -> ("error out"=w8:errorcluster)  [unwired: 9 in]
  n130 = call "Close.vi"("error in (no error)"=w18, "NetworkStreamWriter in"=w19) -> ("error out"=w9:errorcluster)  [unwired: 9 in]
  n131 = Merge Errors(w9, w8) -> (→"Final error out":errorcluster)
